vi "test_Set PCL Decimation.vi"(8 "error in (no error)":errorcluster, 11 "TestCase in":refnum<class "Instrument Addon Scripting API Custom Device Unit Tests.lvclass">) -> (0 "error out":errorcluster, 3 "TestCase out":refnum<class "Instrument Addon Scripting API Custom Device Unit Tests.lvclass">)   [LabVIEW 2018, in "Instrument Addon Scripting API Custom Device Unit Tests.lvclass"]
uses:
  Instrument Addon Scripting API Custom Device Unit Tests.lvclass
  <vilib>/addons/_JKI Toolkits/VI Tester/TestCase.llb/TestCase.lvclass
  APIs/Scripting API/Instrument Addon Scripting API.lvlib
  Instrument Addon Scripting API Test Assets/Instrument Addon Scripting API Test Assets.lvclass
  C:/Program Files (x86)/National Instruments/LabVIEW 2018/vi.lib/addons/_JKI Toolkits/VI Tester/TestCase.llb/TestCase.lvclass
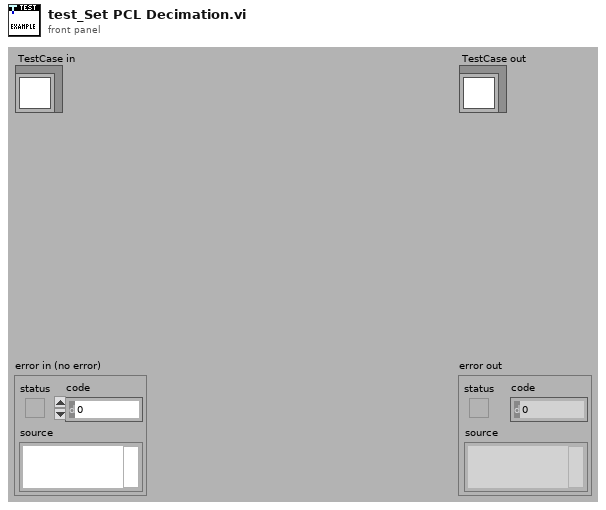
[diagram p1: front panel]
types:
  T1 = typedef "Custom Device API.lvlib/Custom Device Item Ref.ctl" = u64
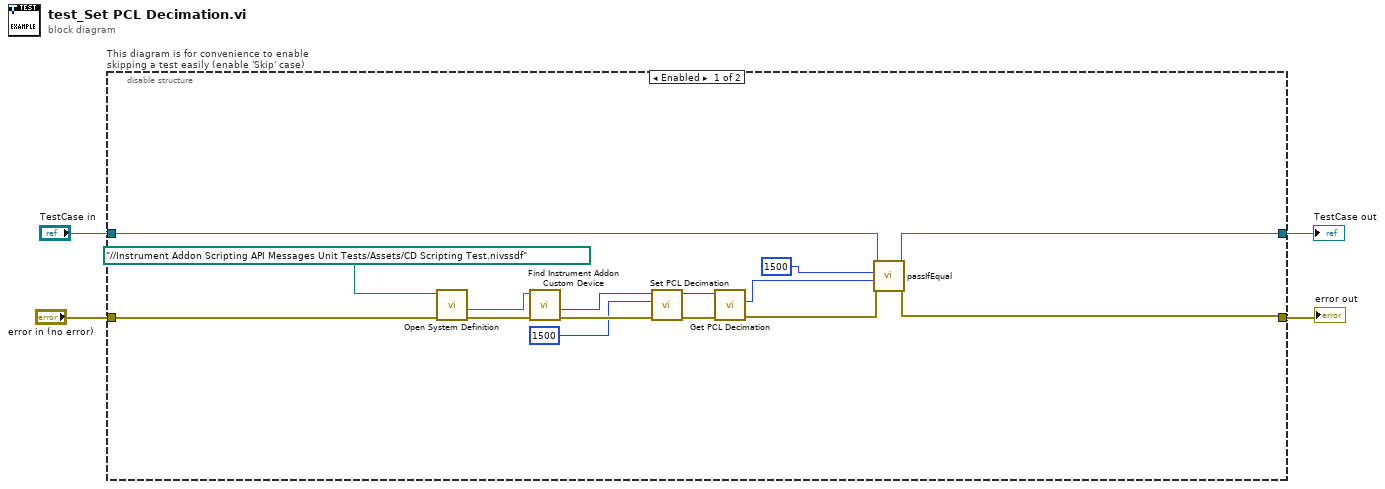
[diagram p0: block diagram]
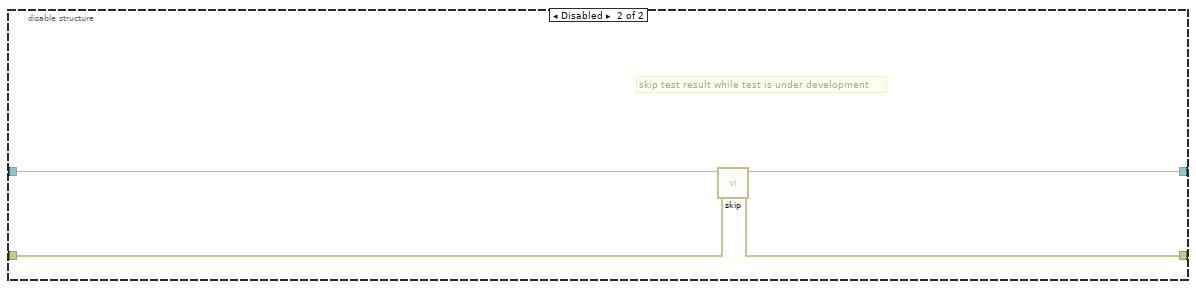
[diagram p2: hidden frame]
diagram:
  n1 = disable-structure "This diagram is for convenience to enable skipping a test easily (enable 'Skip' case)" shown="Enabled" {
    disable-tunnel: "TestCase in" -> [w19 w23]
    disable-tunnel: [w18 w21] -> w1
    disable-tunnel: [w17 w22] -> w3
    disable-tunnel: "error in (no error)" -> [w16 w20]
    frame Enabled {
      n2 = call "Open System Definition.vi"("error in (no error)"=w16, "System Definition File"=path "../../Instrument Addon Scripting API Messages Unit Tests/Assets/CD Scripting Test.nivssdf") -> ("error out"=w14:errorcluster, "Target Refnum"=w13:refnum<k24>)  [unwired: 6 in, 2 out]
      n3 = call "Find Instrument Addon Custom Device.vi"("error in"=w14, "target in"=w13) -> ("error out"=w11:errorcluster, "NodeID"=w12:u64)  [unwired: 7 in, 1 out]
      n4 = call "Set PCL Decimation.vi"("Error In"=w11, "PCL Decimation"=u32 1500, "Instrument Addon Refnum In"=w12) -> ("Error Out"=w9:errorcluster, "Instrument Addon Refnum Out"=w8:T1)  [unwired: 7 in]
      n5 = call "Get PCL Decimation.vi"("Error In"=w9, "Instrument Addon Refnum In"=w8) -> ("Error Out"=w7:errorcluster, "PCL Decimation"=w6:u32)  [unwired: 7 in, 1 out]
      n6 = call-dynamic "passIfEqual.vi"("error in (no error)"=w7, "y"=w6, "x"=u32 1500 ("PCL Decimation"), "TestCase in"=w19) -> ("error out"=w17:errorcluster, "TestCase out"=w18:refnum<class "Instrument Addon Scripting API Custom Device Unit Tests.lvclass">)  [unwired: 6 in]
    }
    frame Disabled {
      # "skip test result while test is under development"
      n7 = call <vilib>:"skip.vi"("error in (no error)"=w20, "TestCase in"=w23) -> ("error out"=w22:errorcluster, "TestCase out"=w21:refnum<class "Instrument Addon Scripting API Custom Device Unit Tests.lvclass">)  [unwired: 8 in]
    }
  }
  "error out" <- w3
  "TestCase out" <- w1
